vi "Set properties lockin.vi"(8 "error in (no error)":errorcluster, 11 "Lockin and Fluke Multimeter in":refnum<class "Lockin and Fluke Multimeter.lvclass">) -> (0 "error out":errorcluster, 3 "Lockin and Fluke Multimeter out":refnum<class "Lockin and Fluke Multimeter.lvclass">)   [LabVIEW 2017, in "Lockin and Fluke Multimeter.lvclass"]
uses:
  Lockin and Fluke Multimeter.lvclass
  Lockin and Fluke Multimeter.lvclass/Lockin and Fluke Multimeter.ctl
  Lockin/sr830/SR830.lvlib
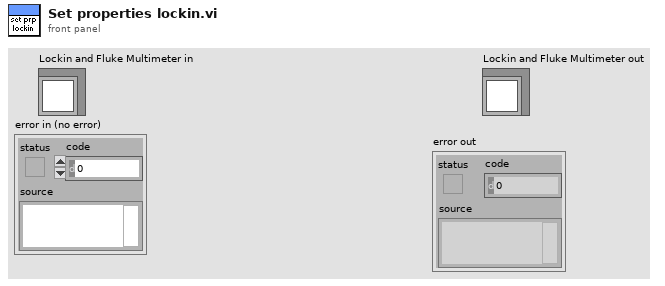
[diagram p1: front panel]
types:
  T1 = typedef "Lockin SR830.lvclass/Sensitivity.ctl" = u16
  T2 = typedef "SR830.lvlib/Tau.ctl" = u16
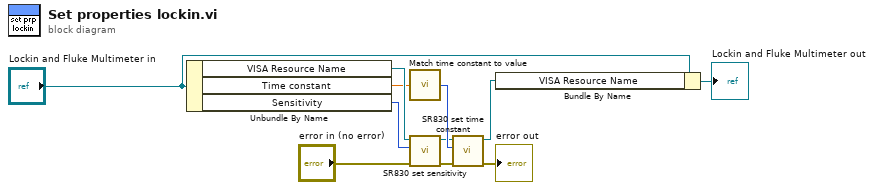
[diagram p0: block diagram]
diagram:
  n1 = Unbundle By Name("Lockin and Fluke Multimeter in") -> ("VISA Resource Name"=w11:refnum<visa-resource-name>, "Time constant"=w7:dbl[unit], "Sensitivity"=w4:T1)
  n2 = call "Match time constant to value.vi"("Time constant"=w7) -> ("Tau"=w6:T2)
  n3 = call "SR830 set sensitivity.vi"("error in (no error)"="error in (no error)", "Sensitivity"=w4, "VISA resource name"=w11) -> ("error out"=w9:errorcluster, "VISA resource name out"=w5:refnum<visa-resource-name>)  [unwired: 7 in]
  n4 = call "SR830 set time constant.vi"("error in (no error)"=w9, "Tau"=w6, "VISA resource name"=w5) -> ("error out"=→"error out":errorcluster, "VISA resource name out"=w2:refnum<visa-resource-name>)  [unwired: 7 in]
  n5 = Bundle By Name(cluster="Lockin and Fluke Multimeter in", "VISA Resource Name"=w2) -> (→"Lockin and Fluke Multimeter out":refnum<class "Lockin and Fluke Multimeter.lvclass">)
